vi "UnscentedKalmanFilter_Correct.vi"(6 "UNSCENTED_KALMAN_CORRECT_FUNC_GROUP":T1, 7 "Rows":i32, 8 "R":T3, 9 "Y":T3, 10 "U":T3, 11 "in UnscentedKalmanFiilter":T4) -> (0 "Error":bool, 3 "out UnscentedKalmanFiilter":T4)   [LabVIEW 2019, in "Trajectory_Library.lvlib"]
doc: "Creates a new LINEAR SYSTEM data cluster with the specified values. \n\n\nInputs: \n - XXX -- XXX.\n\nOutputs:\n - XXX -- XXX."
uses:
  Trajectory_Library.lvlib
  UNSCENTED_KALMAN_FILTER.ctl
  <vilib>/Analysis/Matrix/Datatypes/RealMatrix.ctl
  MERWE_SCALED_SIGMA_PTS.ctl
  BiFun_Matrix_FUNC_TYPE.ctl
  UNSCENTED_KALMAN_CORRECT_FUNC_GROUP.ctl
  <vilib>/Analysis/7linalg.llb/Real Transpose Matrix.vi
  <vilib>/Analysis/baseanly.llb/Real A x B.vi
  <vilib>/Analysis/Matrix/Numeric/Add/Add - RM,RM.vi
  <vilib>/Analysis/Matrix/Numeric/Multiply/Multiply - RM,R.vi
  <vilib>/Analysis/7linalg.llb/Solve Linear Equations (multiple right hand).vi
  <vilib>/Analysis/Matrix/Numeric/Subtract/Subtract - RM,RM.vi
  <vilib>/Analysis/Matrix/NI_Matrix.lvlib
  <vilib>/Analysis/NI_AALPro.lvlib
  <vilib>/Analysis/NI_AALBase.lvlib
panel:
  # "<Inputs, 1>"
  # "<Rows, 1>"
  # "<Rows, Rows>"
  # "State Estimate <Statess,1>"
  # "<States, States>"
  # "<States, ?>"
  # "<Statess,  States>"
  # "<Outputs, Outputs>"
  # "<?, 1>"
  # "<?, 1>"
  # "State Estimate <Statess,1>"
  # "<States, States>"
  # "<States, ?>"
  # "<Statess,  States>"
  # "<Outputs, Outputs>"
  # "<?, 1>"
  # "<?, 1>"
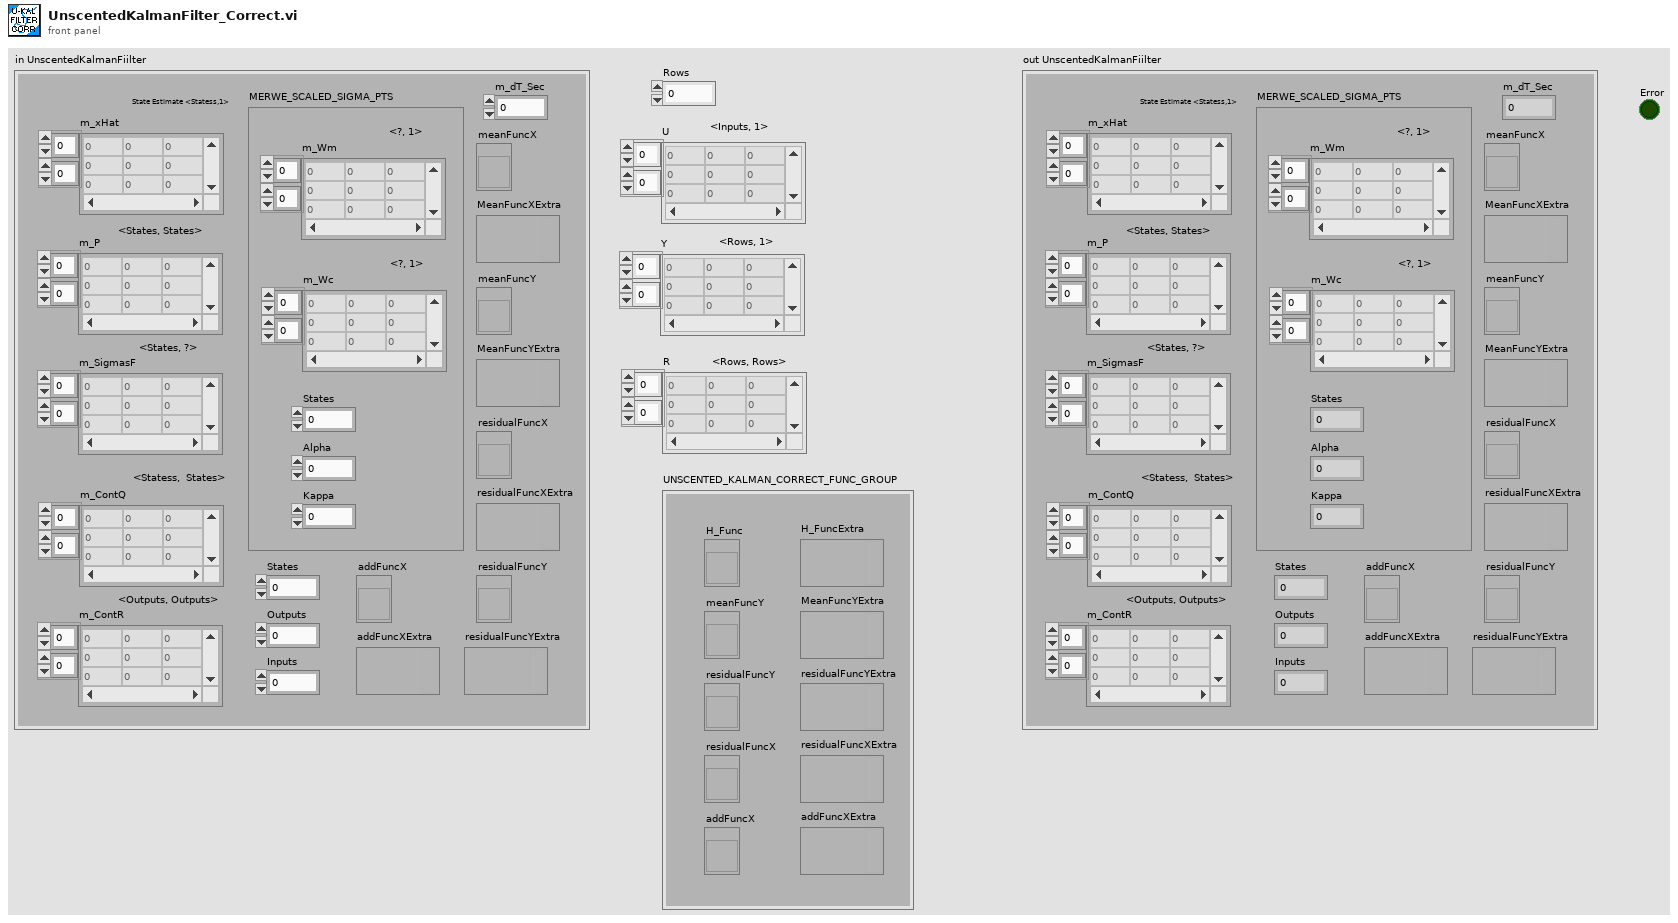
[diagram p1: front panel]
types:
  T1 = typedef "Trajectory_Library.lvlib/UNSCENTED_KALMAN_CORRECT_FUNC_GROUP.ctl" = cluster{"H_Func":T2, "meanFuncY":T2, "residualFuncY":T2, "residualFuncX":T2, "addFuncX":T2, "H_FuncExtra":variant, "MeanFuncYExtra":variant, "residualFuncYExtra":variant, "residualFuncXExtra":variant, "addFuncXExtra":variant}
  T2 = typedef "Trajectory_Library.lvlib/BiFun_Matrix_FUNC_TYPE.ctl" = refnum<vi>
  T3 = typedef "NI_Matrix.lvlib/RealMatrix.ctl" = dbl[][]
  T4 = typedef "Trajectory_Library.lvlib/UNSCENTED_KALMAN_FILTER.ctl" = cluster{"m_P":T3, "m_xHat":T3, "States":i32, "Outputs":i32, "m_ContR":T3, "m_ContQ":T3, "m_SigmasF":T3, "m_dT_Sec":dbl, "MERWE_SCALED_SIGMA_PTS":T5, "meanFuncX":T2, "meanFuncY":T2, "residualFuncX":T2, "residualFuncY":T2, "addFuncX":T2, "addFuncXExtra":variant, "residualFuncYExtra":variant, "residualFuncXExtra":variant, "MeanFuncYExtra":variant, "MeanFuncXExtra":variant, "Inputs":i32}
  T5 = typedef "Trajectory_Library.lvlib/MERWE_SCALED_SIGMA_PTS.ctl" = cluster{"m_Wm":T3, "States":i32, "Alpha":dbl, "m_Wc":T3, "Kappa":i32}
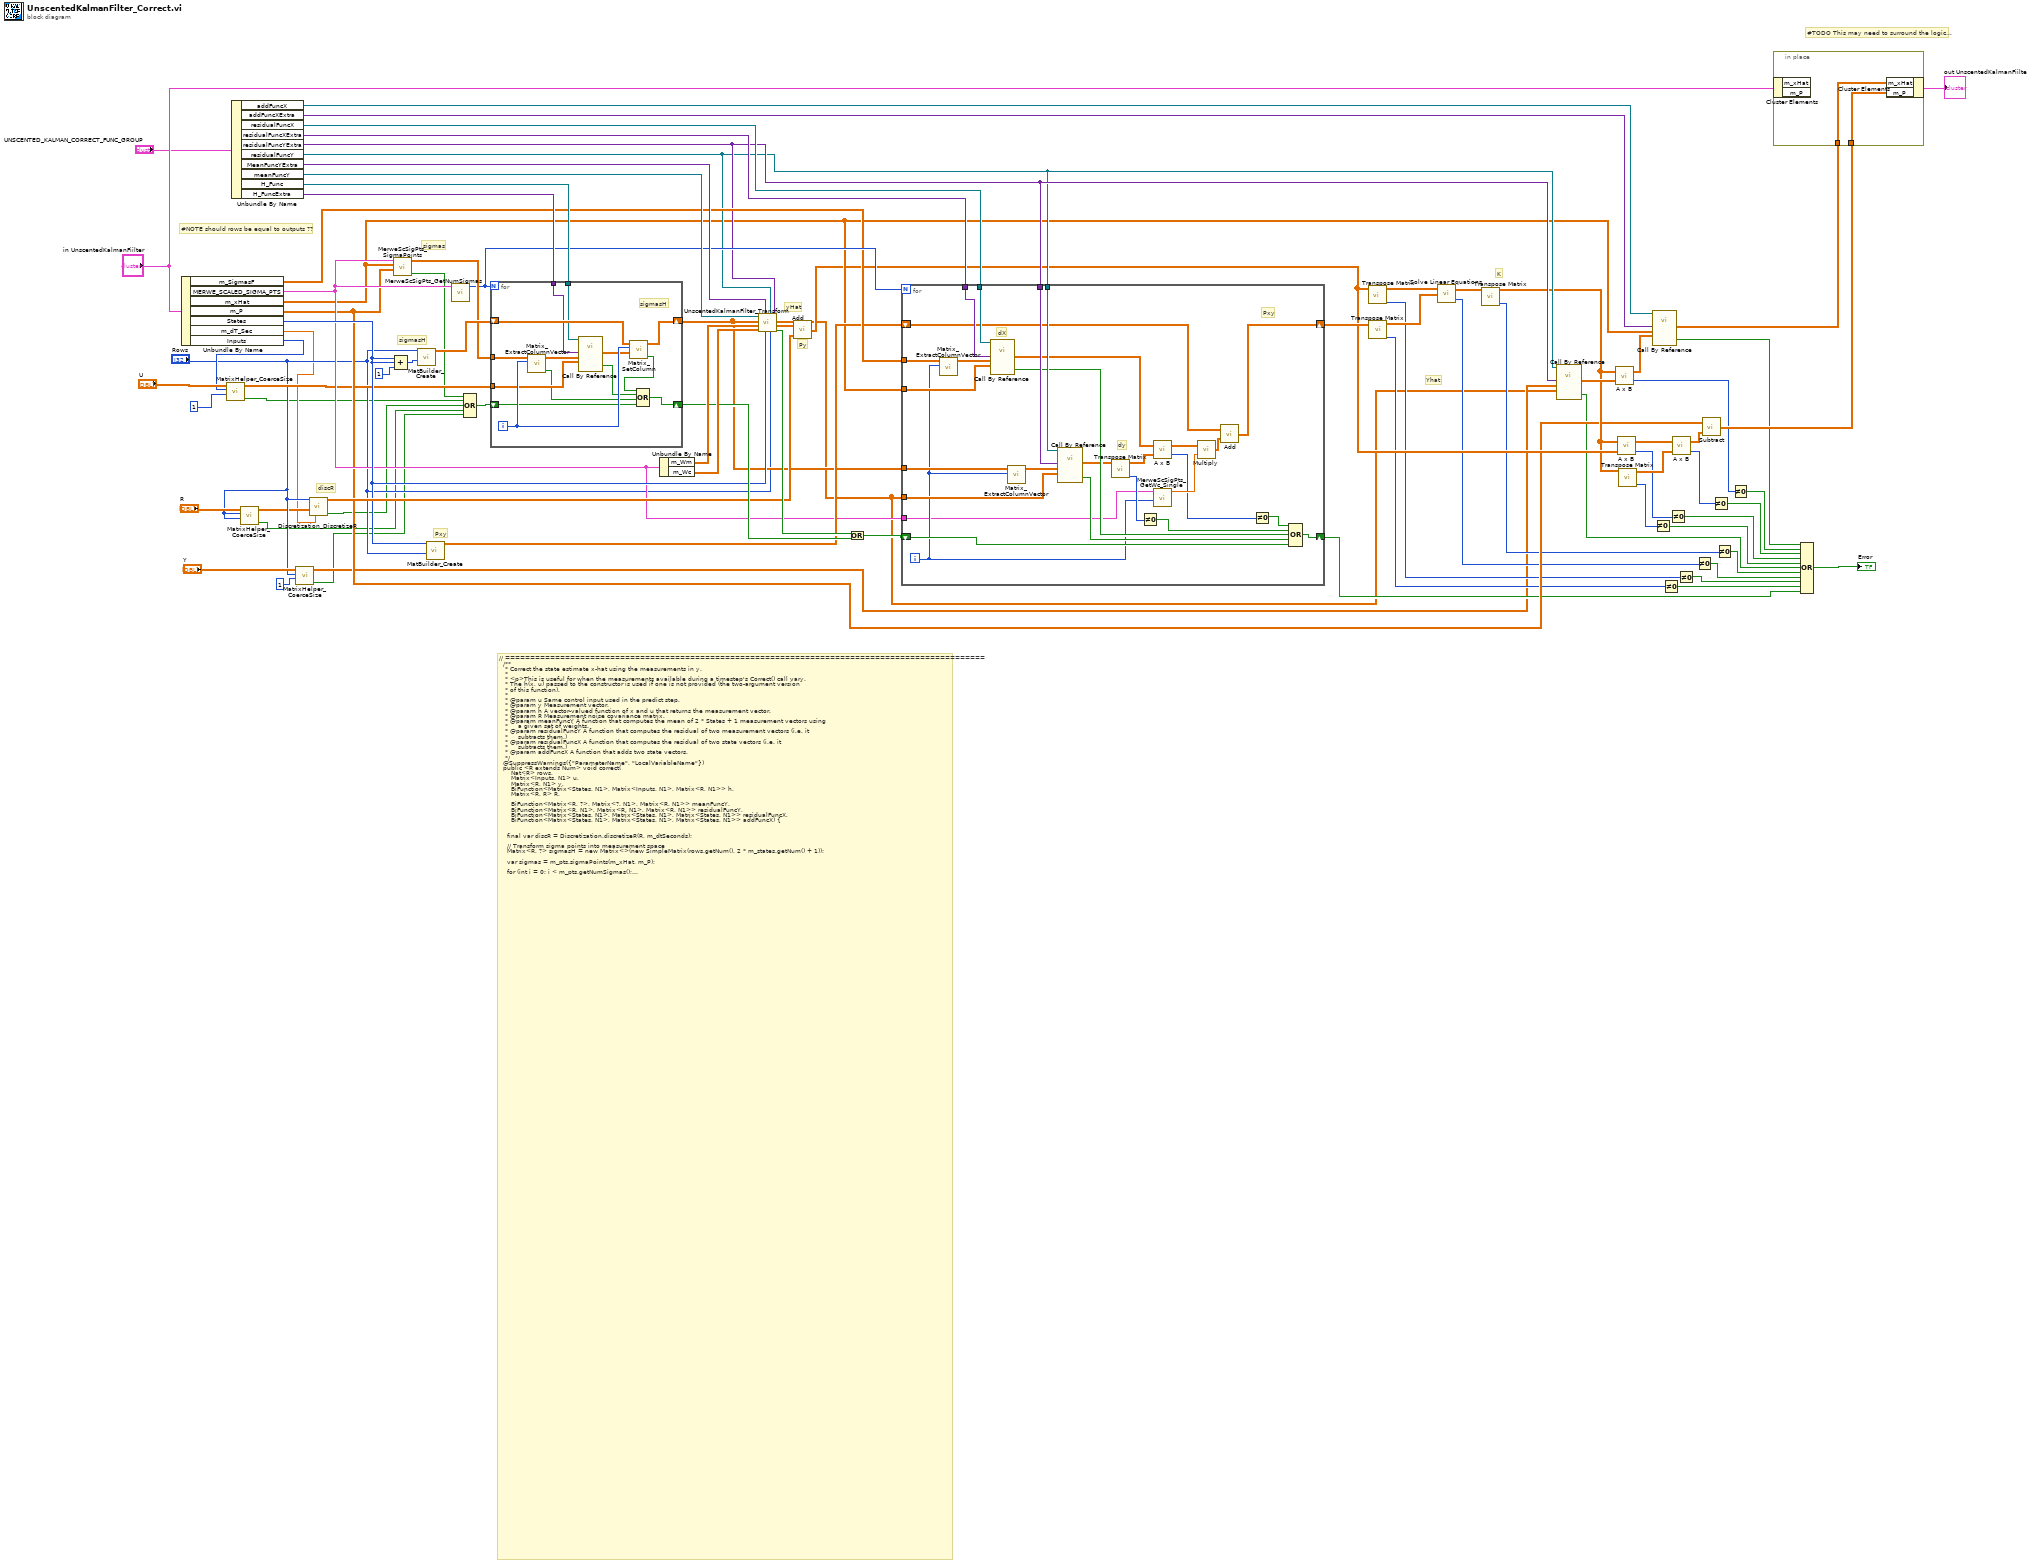
[diagram p0: block diagram]
diagram:
  # "Yhat"
  # "#NOTE should rows be equal to outputs ??"
  # "// ================================================================================================\n  /**\n   * Correct the state estimate x-hat using the measurements in y.\n   *\n   * <p>This is useful for when the measurements available during a timestep's Correct() call vary.\n   * The h(x, u) passed to the constructor is used if one is not provided (the two-argument version\n   * of this function).\n   *\n   * @param u Same control input used in the predict step.\n   * @param y Measurement vector.\n   * @param h A vector-valued function of x and u that returns the measurement vector.\n   * @param R Measurement noise covariance matrix.\n   * @param meanFuncY A function that computes the mean of 2 * States + 1 measurement vectors using\n   *     a given set of weights.\n   * @param residualFuncY A function that computes the residual of two measurement vectors (i.e. it\n   *     subtracts them.)\n   * @param residualFuncX A function that computes the residual of two state vectors (i.e. it\n   *     subtracts them.)\n   * @param addFuncX A function that adds two state vectors.\n   */\n  @SuppressWarnings({\"ParameterName\", \"LocalVariableName\"})\n  public <R extends Num> void correct(\n      Nat<R> rows,\n      Matrix<Inputs, N1> u,\n      Matrix<R, N1> y,\n      BiFunction<Matrix<States, N1>, Matrix<Inputs, N1>, Matrix<R, N1>> h,\n      Matrix<R, R> R,\n\n      BiFunction<Matrix<R, ?>, Matrix<?, N1>, Matrix<R, N1>> meanFuncY,\n      BiFunction<Matrix<R, N1>, Matrix<R, N1>, Matrix<R, N1>> residualFuncY,\n      BiFunction<Matrix<States, N1>, Matrix<States, N1>, Matrix<States, N1>> residualFuncX,\n      BiFunction<Matrix<States, N1>, Matrix<States, N1>, Matrix<States, N1>> addFuncX) {\n\n\n    final var discR = Discretization.discretizeR(R, m_dtSeconds);\n\n    // Transform sigma points into measurement space\n    Matrix<R, ?> sigmasH = new Matrix<>(new SimpleMatrix(rows.getNum(), 2 * m_states.getNum() + 1));\n\n    var sigmas = m_pts.sigmaPoints(m_xHat, m_P);\n\n    for (int i = 0; i < m_pts.getNumSigmas(); i++) {\n      Matrix<R, N1> hRet = h.apply(\n\t\t\tsigmas.extractColumnVector(i), \n\t\t\tu);\n      sigmasH.setColumn(i, hRet);\n    }\n\n    // Mean and covariance of prediction passed through unscented transform\n    var transRet = unscentedTransform(\n            \tm_states, \n\t\trows, \n\t\tsigmasH, \n\t\tm_pts.getWm(), \n\t\tm_pts.getWc(), \n\t\tmeanFuncY, \n\t\tresidualFuncY);\n\n    var yHat = transRet.getFirst();\n\n    var Py = transRet.getSecond().plus(discR);\n\n    // Compute cross covariance of the state and the measurements\n    Matrix<States, R> Pxy = new Matrix<>(m_states, rows);\n\n    for (int i = 0; i < m_pts.getNumSigmas(); i++) {\n\n      // Pxy += (sigmas_f[:, i] - xHat) * (sigmas_h[:, i] - yHat)^T * W_c[i]\n      var dx = residualFuncX.apply(\n\t\tm_sigmasF.extractColumnVector(i), \n\t\tm_xHat);\n\n      var dy = residualFuncY.apply(\n\t\tsigmasH.extractColumnVector(i), \n\t\tyHat)\n\t\t\t.transpose();\n\n      Pxy = Pxy\n\t\t.plus(\n\t\t\tdx.times(dy)\n\t\t\t\t.times(m_pts.getWc(i)));\n    }\n\n    // K = P_{xy} Py^-1\n    // K^T = P_y^T^-1 P_{xy}^T\n    // P_y^T K^T = P_{xy}^T\n    // K^T = P_y^T.solve(P_{xy}^T)\n    // K = (P_y^T.solve(P_{xy}^T)^T\n    Matrix<States, R> K = new Matrix<>(Py.transpose().solve(Pxy.transpose()).transpose());\n\n    // xHat + K * (y - yHat)\n    m_xHat = addFuncX.apply(\n\t\tm_xHat, \n\t\tK.times(\n\t\t\tresidualFuncY.apply(\n\t\t\t\ty, \n\t\t\t\tyHat)));\n    \n    m_P = m_P.minus(\n\t\tK.times(Py)\n\t\t\t.times(K.transpose()));\n  }\n}"
  # "#TODO This may need to surround the logic..."
  # "K"
  # "discR"
  # "Py"
  # "Pxy"
  # "yHat"
  # "sigmasH"
  # "sigmas"
  n1 = Unbundle By Name("in UnscentedKalmanFiilter") -> ("m_SigmasF"=w64:T3, "MERWE_SCALED_SIGMA_PTS"=w58:T5, "m_xHat"=w49:T3, "m_P"=w40:T3, "States"=w66:i32, "m_dT_Sec"=w5:dbl, "Inputs"=w15:i32)
  n2 = call "MatrixHelper_CoerceSize.vi"("Columns"=1, "Rows"=w15, "input matrix"="U") -> ("Coerced"=w1:bool, "output matrix"=w18:T3)  [unwired: 7 in]
  n3 = Unbundle By Name("UNSCENTED_KALMAN_CORRECT_FUNC_GROUP") -> ("addFuncX"=w47:T2, "addFuncXExtra"=w48:variant, "residualFuncX"=w62:T2, "residualFuncXExtra"=w63:variant, "residualFuncYExtra"=w53:variant, "residualFuncY"=w52:T2, "MeanFuncYExtra"=w71:variant, "meanFuncY"=w72:T2, "H_Func"=w76:T2, "H_FuncExtra"=w75:variant)
  n4 = call "MatrixHelper_CoerceSize.vi"("Columns"="Rows", "Rows"="Rows", "input matrix"="R") -> ("Coerced"=w2:bool, "output matrix"=w9:T3)  [unwired: 7 in]
  n5 = call "MatrixHelper_CoerceSize.vi"("Columns"=1, "Rows"="Rows", "input matrix"="Y") -> ("Coerced"=w6:bool, "output matrix"=w14:T3)  [unwired: 7 in]
  n6 = call "Discretization_DiscretizeR.vi"("dT_Seconds"=w5, "ContR"=w9, "Outputs"="Rows") -> ("Size Coerced"=w4:bool, "DiscR"=w67:T3)  [unwired: 7 in]
  n7 = call "MerweScSigPts_SigmaPoints.vi"("P"=w40, "X"=w49, "MerweScaledSigmaPts"=w58) -> ("Error"=w3:bool, "SigmaPoints"=w77:T3)  [unwired: 7 in]
  n8 = Compound Arithmetic op=ADD(w66, w66, 1 ("value")) -> (w80:i32)
  n9 = call "MatBuilder_Create.vi"("Columns"=w80, "Rows"="Rows") -> ("output matrix"=w79:T3)  [unwired: 9 in]
  n10 = call "MatBuilder_Create.vi"("Columns"="Rows", "Rows"=w66) -> ("output matrix"=w61:T3)  [unwired: 9 in]
  n11 = call "MerweScSigPts_GetNumSigmas.vi"("MerweScaledSigmaPts"=w58) -> ("NumSigmas"=w65:i32)  [unwired: 10 in]
  n12 = Compound Arithmetic op=OR(w3, w1, w4, w2, w6) -> (w7:bool)
  n13 = for {
    N: w65 -> [_]
    shift-right: [w97] -> w60
    shift-left: w79 -> [w94]
    shift-right: [w95] -> w69
    shift-left: w7 -> [w88]
    tunnel: w77 -> [w93]
    tunnel: w76 -> [w92]
    tunnel: w75 -> [w91]
    tunnel: w18 -> [w89]
    i -> [w96]
    # "sigmasH"
    n14 = call "Matrix_ExtractColumnVector.vi"("Column"=w96, "input matrix"=w93) -> ("Error"=w84:bool, "output column"=w90:T3)  [unwired: 8 in]
    n15 = call-by-ref "?"(reference=w92, "U"=w89, "X"=w90, "Variant"=w91) -> ("Error"=w86:bool, "NewX"=w87:T3)  [unwired: 8 in, 2 out]
    n16 = call "Matrix_SetColumn.vi"("Fill Vector"=w87, "Column"=w96, "input matrix"=w94) -> ("Error"=w85:bool, "output matrix"=w97:T3)  [unwired: 7 in]
    n17 = Compound Arithmetic op=OR(w85, w86, w84, w88) -> (w95:bool)
  }
  n18 = Unbundle By Name(w58) -> ("m_Wm"=w74:T3, "m_Wc"=w73:T3)
  n19 = call "UnscentedKalmanFilter_Transform.vi"("ResidualFuncExtra"=w53, "Dim"="Rows", "residualFunc"=w52, "S"=w66, "MeanFuncExtra"=w71, "Wc"=w73, "Wm"=w74, "Sigmas"=w60, "MeanFunc"=w72) -> ("Error"=w70:bool, "P"=w68:T3, "X"=w8:T3)
  n20 = call-poly <vilib>:"Add.vi"("Real Matrix B"=w67, "Real Matrix A"=w68) -> ("A + B"=w45:T3)
  n21 = Or(x=w70, y=w69) -> (x .or. y?=w59:bool)
  n22 = for {
    N: w65 -> [_]
    shift-right: [w100] -> w57
    shift-left: w61 -> [w101]
    shift-right: [w125] -> w34
    shift-left: w59 -> [w119]
    tunnel: w64 -> [w124]
    tunnel: w62 -> [w123]
    tunnel: w63 -> [w122]
    tunnel: w49 -> [w120]
    tunnel: w53 -> [w117]
    tunnel: w52 -> [w116]
    tunnel: w60 -> [w115]
    tunnel: w8 -> [w114]
    tunnel: w58 -> [w105]
    i -> [w106]
    # "Pxy"
    # "dy"
    # "dX"
    n23 = call "Matrix_ExtractColumnVector.vi"("Column"=w106, "input matrix"=w124) -> ("output column"=w121:T3)  [unwired: 8 in, 1 out]
    n24 = call-by-ref "?"(reference=w123, "U"=w120, "X"=w121, "Variant"=w122) -> ("Error"=w113:bool, "NewX"=w107:T3)  [unwired: 8 in, 2 out]
    n25 = call "Matrix_ExtractColumnVector.vi"("Column"=w106, "input matrix"=w115) -> ("output column"=w118:T3)  [unwired: 8 in, 1 out]
    n26 = call-by-ref "?"(reference=w116, "U"=w114, "X"=w118, "Variant"=w117) -> ("Error"=w112:bool, "NewX"=w111:T3)  [unwired: 8 in, 2 out]
    n27 = call-poly <vilib>:"Transpose Matrix.vi"("Input Matrix"=w111) -> ("error"=w109:i32, "Matrix Transpose"=w108:T3)  [unwired: 9 in]
    n28 = Not Equal To 0?(x=w109) -> (x != 0?=w110:bool)
    n29 = call-poly <vilib>:"A x B.vi"("B"=w108, "A"=w107) -> ("error"=w102:i32, "A x B"=w103:T3)
    n30 = call "MerweScSigPts_GetWc_Single.vi"("Element"=w106, "MerweScaledSigmaPts"=w105) -> ("Wc_Value"=w104:dbl)  [unwired: 9 in]
    n31 = call-poly <vilib>:"Multiply.vi"("Real Scalar c"=w104, "Real Matrix A"=w103) -> ("A * c"=w99:T3)
    n32 = call-poly <vilib>:"Add.vi"("Real Matrix B"=w99, "Real Matrix A"=w101) -> ("A + B"=w100:T3)
    n33 = Not Equal To 0?(x=w102) -> (x != 0?=w98:bool)
    n34 = Compound Arithmetic op=OR(w98, w110, w113, w112, w119) -> (w125:bool)
  }
  n35 = call-poly <vilib>:"Transpose Matrix.vi"("Input Matrix"=w45) -> ("error"=w37:i32, "Matrix Transpose"=w56:T3)  [unwired: 9 in]
  n36 = call-poly <vilib>:"Transpose Matrix.vi"("Input Matrix"=w57) -> ("error"=w38:i32, "Matrix Transpose"=w55:T3)  [unwired: 9 in]
  n37 = call-poly <vilib>:"Solve Linear Equations.vi"("Known Matrix"=w55, "Input Matrix"=w56) -> ("error"=w36:i32, "Solution Matrix"=w54:T3)  [unwired: 1 in]
  n38 = call-poly <vilib>:"Transpose Matrix.vi"("Input Matrix"=w54) -> ("error"=w35:i32, "Matrix Transpose"=w44:T3)  [unwired: 9 in]
  n39 = call-by-ref "?"(reference=w52, "U"=w8, "X"=w14, "Variant"=w53) -> ("Error"=w29:bool, "NewX"=w51:T3)  [unwired: 8 in, 2 out]
  n40 = call-poly <vilib>:"A x B.vi"("B"=w51, "A"=w44) -> ("error"=w25:i32, "A x B"=w50:T3)
  n41 = call-poly <vilib>:"A x B.vi"("B"=w45, "A"=w44) -> ("error"=w27:i32, "A x B"=w43:T3)
  n42 = call-poly <vilib>:"Transpose Matrix.vi"("Input Matrix"=w44) -> ("error"=w28:i32, "Matrix Transpose"=w42:T3)  [unwired: 9 in]
  n43 = call-by-ref "?"(reference=w47, "U"=w50, "X"=w49, "Variant"=w48) -> ("Error"=w20:bool, "NewX"=w46:T3)  [unwired: 8 in, 2 out]
  n44 = Not Equal To 0?(x=w28) -> (x != 0?=w24:bool)
  n45 = Not Equal To 0?(x=w38) -> (x != 0?=w33:bool)
  n46 = Not Equal To 0?(x=w27) -> (x != 0?=w23:bool)
  n47 = call-poly <vilib>:"A x B.vi"("B"=w42, "A"=w43) -> ("error"=w26:i32, "A x B"=w41:T3)
  n48 = Not Equal To 0?(x=w37) -> (x != 0?=w32:bool)
  n49 = Not Equal To 0?(x=w36) -> (x != 0?=w31:bool)
  n50 = call-poly <vilib>:"Subtract.vi"("Real Matrix B"=w41, "Real Matrix A"=w40) -> ("A - B"=w39:T3)
  n51 = Not Equal To 0?(x=w26) -> (x != 0?=w22:bool)
  n52 = Not Equal To 0?(x=w35) -> (x != 0?=w30:bool)
  n53 = Not Equal To 0?(x=w25) -> (x != 0?=w21:bool)
  n54 = in-place {
    in-place-border: w46 -> [w127]
    in-place-border: w39 -> [w126]
    n55 = in-place-cluster #1("in UnscentedKalmanFiilter") -> ()  [unwired: 2 out]
    n56 = in-place-cluster #1("m_xHat"=w127, "m_P"=w126) -> (→"out UnscentedKalmanFiilter":T4)
  }
  n57 = Compound Arithmetic op=OR(w20, w21, w22, w23, w24, w29, w30, w31, w32, w33, w34) -> (→"Error":bool)
